vi "WriteNumericRegister.vi"(8 "Value":sgl, 9 "index":i32, 10 "Snpx":refnum<k24>, 11 "error in":errorcluster) -> (3 "error out":errorcluster)   [LabVIEW 2018, in "UnderAutomation.Fanuc.lvlib"]
uses:
  UnderAutomation.Fanuc.lvlib
  C:/Users/fg/Documents/Fanuc.vi/LabVIEW_2024/UnderAutomation.Fanuc/lib/UnderAutomation.Fanuc.dll
  LabVIEW_2024/UnderAutomation.Fanuc/lib/UnderAutomation.Fanuc.dll
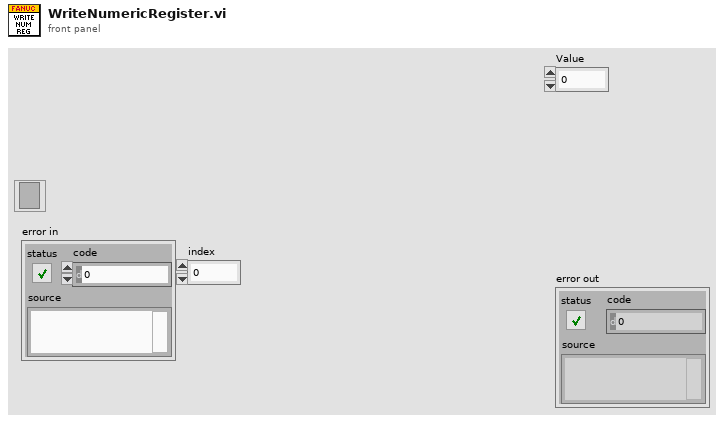
[diagram p1: front panel]
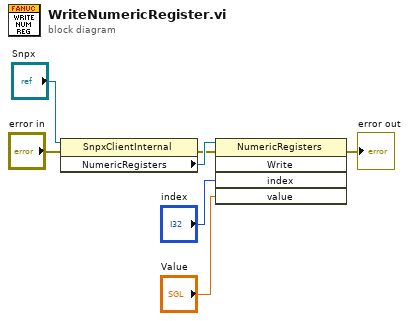
[diagram p0: block diagram]
diagram:
  n1 = property class="SnpxClientInternal"(reference="Snpx", error in="error in") -> (error out=w4:errorcluster, "NumericRegisters"=w5:refnum<k24>)  [unwired: 1 out]
  n2 = invoke class="NumericRegisters" method="Write"(reference=w5, error in=w4, "index"="index", "value"="Value") -> (error out=→"error out":errorcluster)  [unwired: 1 in, 4 out]
